vi "Two Shimmer.vi"() -> ()   [LabVIEW 2025]
uses:
  C:/Github/Shimmer-Labview-API/ShimmerLabview/Bin/ShimmerLVWrapper.dll
  Bin/ShimmerLVWrapper.dll
panel:
  out "Waveform Chart 2":cluster{dbl, dbl, dbl}(graph)
  out "Waveform Chart":cluster{dbl, dbl, dbl}(graph)
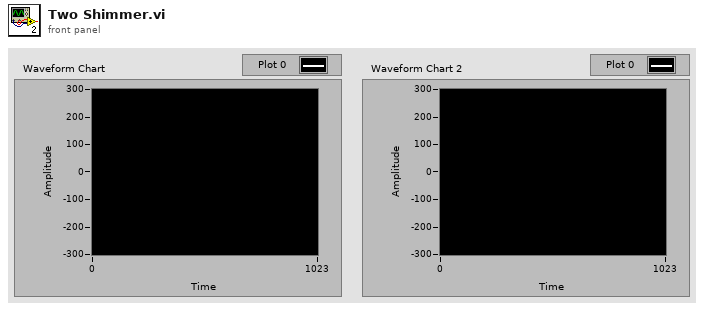
[diagram p1: front panel]
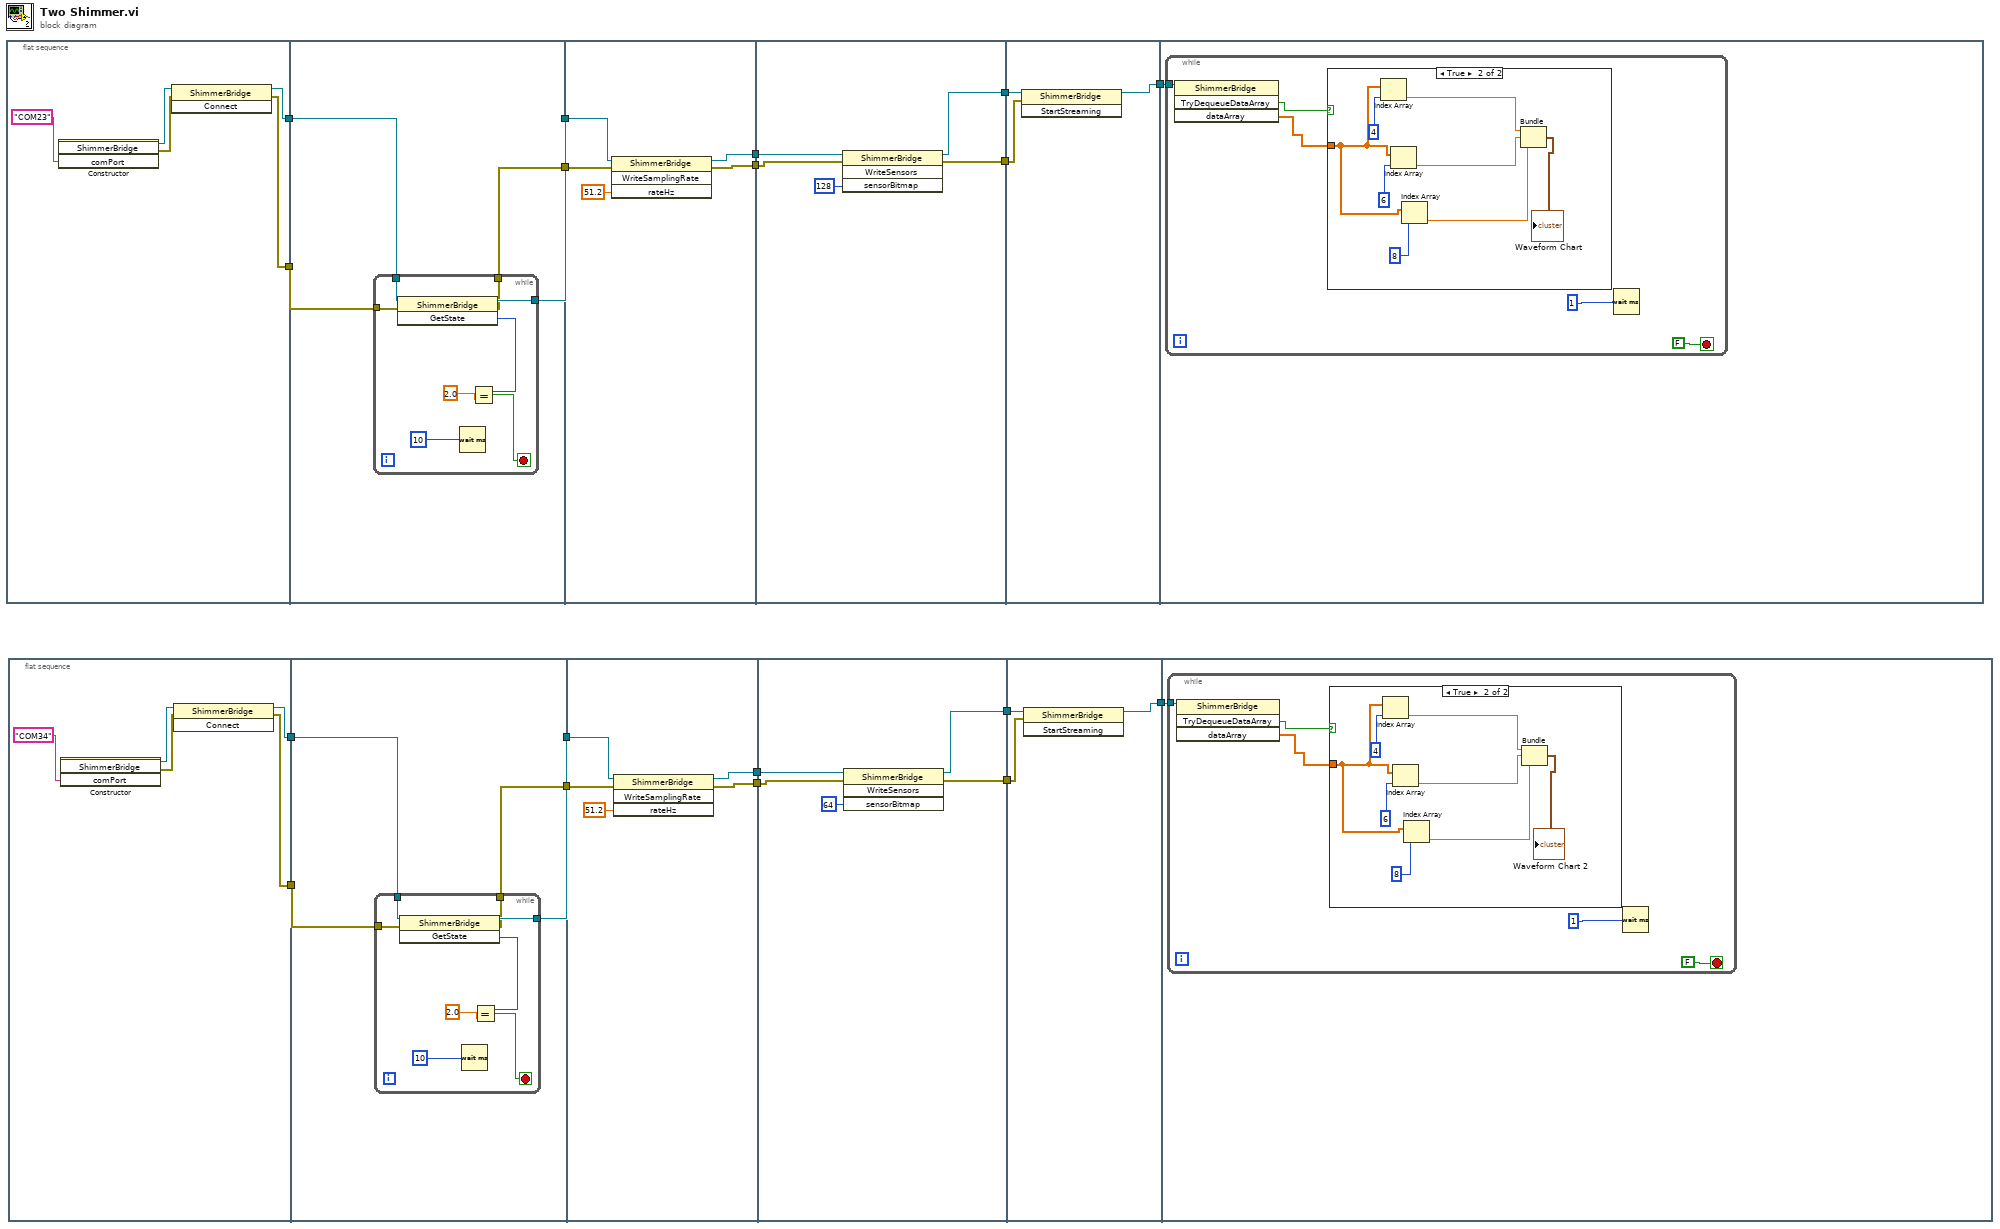
[diagram p0: block diagram]
diagram:
  n1 = flat-sequence {
    tunnel: [w20] -> w18
    tunnel: [w19] -> w17
    tunnel: w18 -> [w27]
    tunnel: [w26] -> w16
    tunnel: w17 -> [w24]
    tunnel: [w25] -> w15
    tunnel: w16 -> [w40]
    tunnel: [w39] -> w14
    tunnel: [w38] -> w13
    tunnel: w15 -> [w36]
    tunnel: w14 -> [w45]
    tunnel: [w44] -> w12
    tunnel: w13 -> [w43]
    tunnel: [w42] -> w11
    tunnel: [w48] -> w10
    tunnel: w12 -> [w47]
    tunnel: w11 -> [w46]
    tunnel: w10 -> [w49]
    frame #0 {
      n2 = constructor class="ShimmerBridge"("comPort"="COM23") -> (reference out=w22:refnum<k24>, error out=w21:errorcluster)  [unwired: 3 in, 2 out]
      n3 = invoke class="ShimmerBridge" method="Connect"(reference=w22, error in=w21) -> (reference out=w20:refnum<k24>, error out=w19:errorcluster)  [unwired: 1 in, 1 out]
    }
    frame #1 {
      n4 = while {
        tunnel: w27 -> [w33]
        tunnel: [w32] -> w26
        tunnel: [w31] -> w25
        tunnel: w24 -> [w30]
        stop <- w35 stop-if-true
        n5 = invoke class="ShimmerBridge" method="GetState"(reference=w33, error in=w30) -> (reference out=w32:refnum<k24>, error out=w31:errorcluster, "GetState"=w29:i32)  [unwired: 1 in]
        n6 = Wait (ms)(milliseconds to wait=u32 10 ("millisecond timer value")) -> ()  [unwired: 1 out]
        n7 = Equal?(x=w29, y=2.0 ("rateHz")) -> (x = y?=w35:bool)
      }
    }
    frame #2 {
      n8 = invoke class="ShimmerBridge" method="WriteSamplingRate"(reference=w40, error in=w36, "rateHz"=51.2) -> (reference out=w39:refnum<k24>, error out=w38:errorcluster)  [unwired: 1 in, 2 out]
    }
    frame #3 {
      n9 = invoke class="ShimmerBridge" method="WriteSensors"(reference=w45, error in=w43, "sensorBitmap"=128) -> (reference out=w44:refnum<k24>, error out=w42:errorcluster)  [unwired: 1 in, 2 out]
    }
    frame #4 {
      n10 = invoke class="ShimmerBridge" method="StartStreaming"(reference=w47, error in=w46) -> (reference out=w48:refnum<k24>)  [unwired: 1 in, 2 out]
    }
    frame #5 {
      n11 = while {
        tunnel: w49 -> [w52]
        stop <- FALSE stop-if-true
        n12 = invoke class="ShimmerBridge" method="TryDequeueDataArray"(reference=w52) -> ("TryDequeueDataArray"=w51:bool, "dataArray"=w50:dbl[])  [unwired: 3 in, 2 out]
        n13 = case shown="True" w51 {
          tunnel: w50 -> [_ w59]
          frame False {
          }
          frame True {
            n14 = Index Array(array=w59, index=4) -> (element=w58:dbl)
            n15 = Index Array(array=w59, index=6) -> (element=w57:dbl)
            n16 = Index Array(array=w59, index=8) -> (element=w56:dbl)
            n17 = Bundle(w58, w57, w56) -> (→"Waveform Chart":cluster{dbl, dbl, dbl})  [unwired: 1 in]
          }
        }
        n18 = Wait (ms)(milliseconds to wait=u32 1) -> ()  [unwired: 1 out]
      }
    }
  }
  n19 = flat-sequence {
    tunnel: [w64] -> w9
    tunnel: [w63] -> w8
    tunnel: w9 -> [w71]
    tunnel: [w70] -> w7
    tunnel: w8 -> [w68]
    tunnel: [w69] -> w6
    tunnel: w7 -> [w84]
    tunnel: [w83] -> w5
    tunnel: [w82] -> w4
    tunnel: w6 -> [w80]
    tunnel: w5 -> [w89]
    tunnel: [w88] -> w3
    tunnel: w4 -> [w87]
    tunnel: [w86] -> w2
    tunnel: [w92] -> w1
    tunnel: w3 -> [w91]
    tunnel: w2 -> [w90]
    tunnel: w1 -> [w93]
    frame #0 {
      n20 = constructor class="ShimmerBridge"("comPort"="COM34") -> (reference out=w66:refnum<k24>, error out=w65:errorcluster)  [unwired: 3 in, 2 out]
      n21 = invoke class="ShimmerBridge" method="Connect"(reference=w66, error in=w65) -> (reference out=w64:refnum<k24>, error out=w63:errorcluster)  [unwired: 1 in, 1 out]
    }
    frame #1 {
      n22 = while {
        tunnel: w71 -> [w77]
        tunnel: [w76] -> w70
        tunnel: [w75] -> w69
        tunnel: w68 -> [w74]
        stop <- w79 stop-if-true
        n23 = invoke class="ShimmerBridge" method="GetState"(reference=w77, error in=w74) -> (reference out=w76:refnum<k24>, error out=w75:errorcluster, "GetState"=w73:i32)  [unwired: 1 in]
        n24 = Wait (ms)(milliseconds to wait=u32 10 ("millisecond timer value")) -> ()  [unwired: 1 out]
        n25 = Equal?(x=w73, y=2.0 ("rateHz")) -> (x = y?=w79:bool)
      }
    }
    frame #2 {
      n26 = invoke class="ShimmerBridge" method="WriteSamplingRate"(reference=w84, error in=w80, "rateHz"=51.2) -> (reference out=w83:refnum<k24>, error out=w82:errorcluster)  [unwired: 1 in, 2 out]
    }
    frame #3 {
      n27 = invoke class="ShimmerBridge" method="WriteSensors"(reference=w89, error in=w87, "sensorBitmap"=64) -> (reference out=w88:refnum<k24>, error out=w86:errorcluster)  [unwired: 1 in, 2 out]
    }
    frame #4 {
      n28 = invoke class="ShimmerBridge" method="StartStreaming"(reference=w91, error in=w90) -> (reference out=w92:refnum<k24>)  [unwired: 1 in, 2 out]
    }
    frame #5 {
      n29 = while {
        tunnel: w93 -> [w96]
        stop <- FALSE stop-if-true
        n30 = invoke class="ShimmerBridge" method="TryDequeueDataArray"(reference=w96) -> ("TryDequeueDataArray"=w95:bool, "dataArray"=w94:dbl[])  [unwired: 3 in, 2 out]
        n31 = case shown="True" w95 {
          tunnel: w94 -> [_ w103]
          frame False {
          }
          frame True {
            n32 = Index Array(array=w103, index=4) -> (element=w102:dbl)
            n33 = Index Array(array=w103, index=6) -> (element=w101:dbl)
            n34 = Index Array(array=w103, index=8) -> (element=w100:dbl)
            n35 = Bundle(w102, w101, w100) -> (→"Waveform Chart 2":cluster{dbl, dbl, dbl})  [unwired: 1 in]
          }
        }
        n36 = Wait (ms)(milliseconds to wait=u32 1) -> ()  [unwired: 1 out]
      }
    }
  }
